vi "GetDataString.vi"(8 "error in (no error)":errorcluster, 11 "FolloWin in":refnum<class "FolloWin.lvclass">) -> (0 "error out":errorcluster, 2 "DataString":string, 3 "FolloWin out":refnum<class "FolloWin.lvclass">)   [LabVIEW 2023, in "FolloWin.lvclass"]
doc: "Gets the DataString from the FolloWin"
uses:
  FolloWin.lvclass
  FolloWin.lvclass/FolloWin.ctl
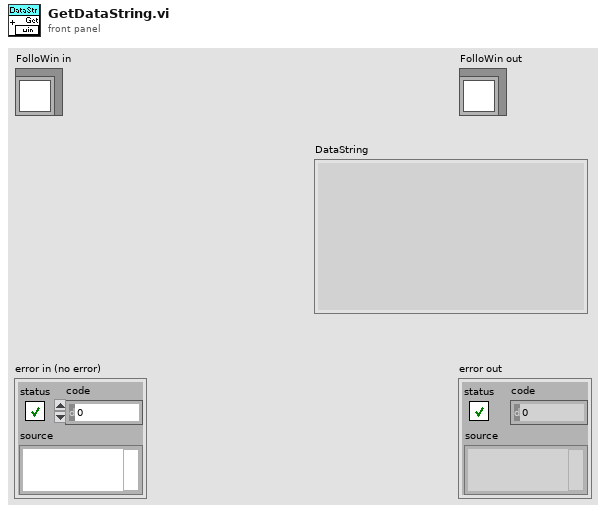
[diagram p1: front panel]
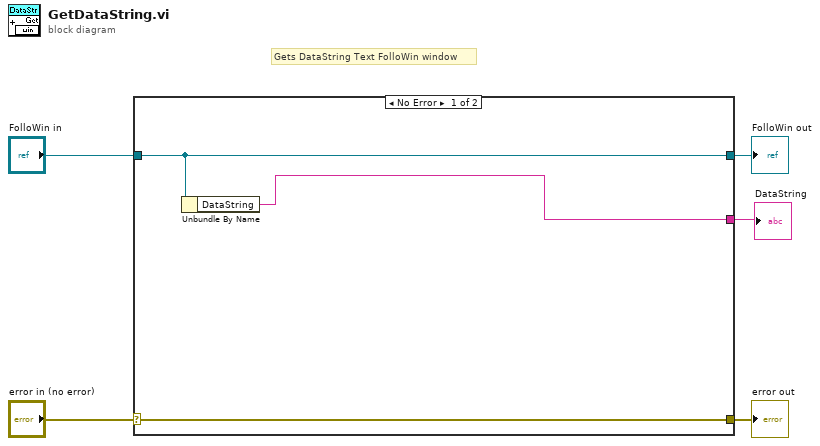
[diagram p0: block diagram]
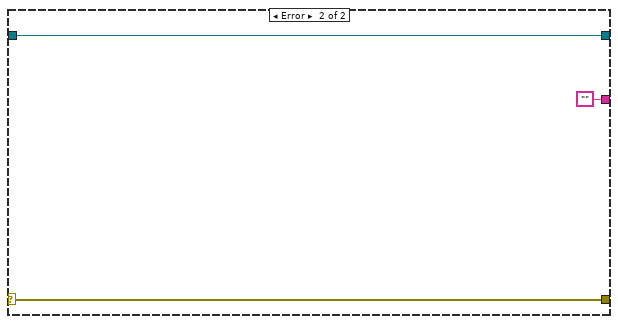
[diagram p2: hidden frame]
diagram:
  # "Gets DataString Text FolloWin window"
  n1 = case shown="No Error" "error in (no error)" {
    selector: "error in (no error)" -> [w6 w11]
    tunnel: [w6 w11] -> w4
    tunnel: [w8 w10] -> w2
    tunnel: "FolloWin in" -> [w8 w10]
    tunnel: [w7 "" ("Value")] -> w1
    frame No Error {
      n2 = Unbundle By Name(w8) -> ("DataString"=w7:string)
    }
    frame Error {
    }
  }
  "error out" <- w4
  "FolloWin out" <- w2
  "DataString" <- w1
